vi "Main.vi"() -> (3 "Angle":dbl format="%#_4g")   [LabVIEW 2021]
doc: "The myRIO Project template acquires acceleration data from the onboard accelerometer and displays the changes of acceleration values in a waveform chart."
uses:
  <vilib>/myRIO/Instrument Drivers/Utilities/Utilities.lvlib
  <vilib>/myRIO/Express VI/Onboard IO/DO/DO Express VI.xnode
  <vilib>/myRIO/Instrument Drivers/Onboard IO/DIO/vis/Write.vi
  <vilib>/myRIO/Instrument Drivers/Onboard IO/DIO/DIO.lvlib
  <vilib>/myRIO/Common/Instrument Driver Framework/myRIO v1.0/DIO/typedefs/DIO Channels Enum.ctl
  <vilib>/myRIO/Common/Instrument Driver Framework/myRIO v1.0/DIO/typedefs/DIO Channels List.ctl
  <vilib>/myRIO/Common/Instrument Driver Framework/Utilities/typedefs/Generic FPGA Reference.ctl
  <vilib>/myRIO/Common/Instrument Driver Framework/Utilities/typedefs/myRIO v1.0 Reference.ctl
  <vilib>/myRIO/Common/Instrument Driver Framework/Utilities/typedefs/Hardware Version Enum.ctl
  <vilib>/myRIO/Common/Instrument Driver Framework/Utilities/typedefs/myRIO Generic Hardware Reference.ctl
  <vilib>/myRIO/Instrument Drivers/Onboard IO/DIO/typedefs/DIO Reference.ctl
  <vilib>/myRIO/Instrument Drivers/Onboard IO/DIO/vis/myRIO DIO Open.xnode
  <vilib>/myRIO/Common/Instrument Driver Framework/Utilities/vis/Is FPGA Ref Available.vi
  <vilib>/myRIO/Common/Instrument Driver Framework/myRIO v1.0/DIO/vis/myRIO v1.1 Open DIO.vi
  <vilib>/userdefined/High Color/nirio_resource_hc.ctl
panel:
  out "Solenoid":bool
  out "Pump":bool
  out "Angle Y":dbl format="%#_4g"
  out "Duty cycle Y":dbl format="%#_3g"
  in  "Stop Button":bool
  out "Duty cycle":dbl format="%#_3g"
  out "?":errorcluster
  # "Servo X"
  # "Servo Y"
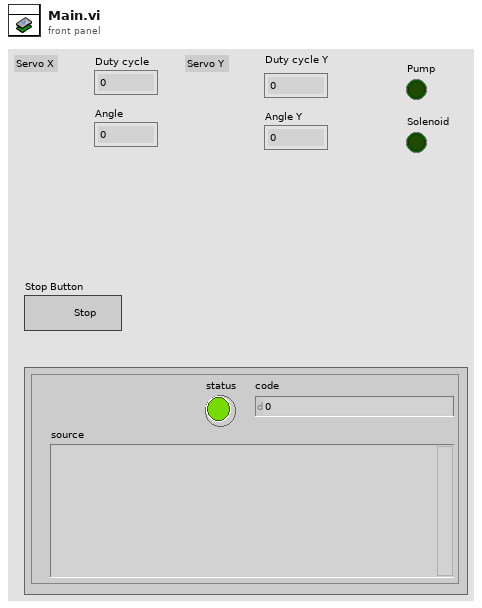
[diagram p1: front panel]
types:
  T1 = typedef "DIO.lvlib/DIO Reference.ctl" = cluster{"myRIO Reference":T2, "DIO Channels List":T6}
  T2 = typedef "myRIO Generic Hardware Reference.ctl" = cluster{"myRIO Model":T3, "myRIO Hardware Reference":T4}
  T3 = typedef "Hardware Version Enum.ctl" = enum16{"Unknown", "myRIO-1900", "myRIO-1950", "roboRIO", "NI ELVIS RIO CM", "ELVIS III"}
  T4 = typedef "myRIO v1.0 Reference.ctl" = cluster{"Generic FPGA Reference":T5, "Allow multiple opens":bool}
  T5 = typedef "Generic FPGA Reference.ctl" = refnum<k20>
  T6 = typedef "DIO Channels List.ctl" = T7[]
  T7 = typedef "DIO Channels Enum.ctl" = enum16{"Not Connected", "C/DIO0", "C/DIO1", "C/DIO2", "C/DIO3", "C/DIO4", "C/DIO5", "C/DIO6", "C/DIO7", "A/DIO0", "A/DIO1", "A/DIO2", "A/DIO3", "A/DIO4", "A/DIO5", "A/DIO6", "A/DIO7", "A/DIO8", "A/DIO9", "A/DIO10", "A/DIO11", "A/DIO12", "A/DIO13", "A/DIO14", "A/DIO15", "A/DIO16", "A/DIO17", "A/DIO18", "A/DIO19", "B/DIO0", "B/DIO1", "B/DIO2", "B/DIO3", "B/DIO4", "B/DIO5", "B/DIO6", "B/DIO7", "B/DIO8", "B/DIO9", "B/DIO10", "B/DIO11", "B/DIO12", "B/DIO13", "B/DIO14", "B/DIO15", "B/DIO16", "B/DIO17", "B/DIO18", "B/DIO19", "LED0", "LED1", "LED2", "LED3", "Button0", "DIO/DIO0", "DIO/DIO1", "DIO/DIO2", "DIO/DIO3", "DIO/DIO4", "DIO/DIO5", "DIO/DIO6", "DIO/DIO7", "DIO/DIO8", "DIO/DIO9", "SPI/CS0", "SPI/CS1", "SPI/CS2", "SPI/CS3", "LED RADIO (Green)", "LED RADIO (Red)", "LED COMM (Green)", "LED COMM (Red)", "LED MODE (Green)", "LED MODE (Red)"}
  T8 = typedef "nirio_resource_hc.ctl" = tag
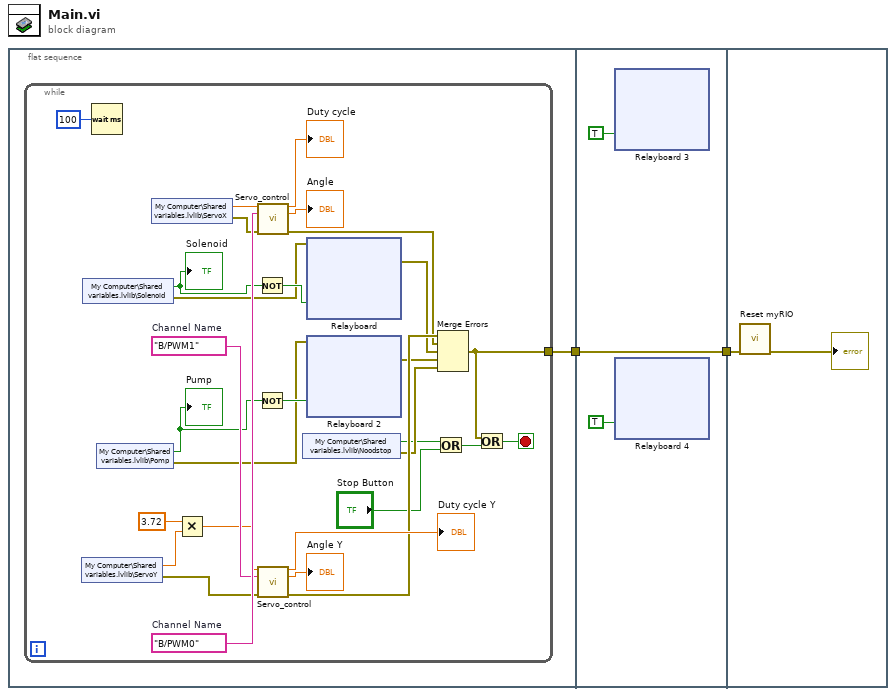
[diagram p0: block diagram]
diagram:
  n1 = flat-sequence {
    tunnel: [w3] -> w2
    tunnel: w2 -> [w105]
    tunnel: [w105] -> w1
    tunnel: w1 -> [w176]
    frame #0 {
      n2 = while {
        tunnel: [w23] -> w3
        stop <- w14 stop-if-true
        w28 = tag "B/PWM1"  # Channel Name
        w29 = tag "B/PWM0"  # Channel Name
        n3 = shared-variable "My Computer\\Shared variables.lvlib\\ServoY"() -> (w6:dbl, error out=w27:errorcluster)  [unwired: 1 in]
        n4 = shared-variable "My Computer\\Shared variables.lvlib\\Solenoid"() -> (w17:bool, error out=w13:errorcluster)  [unwired: 1 in]
        "Solenoid" <- w17
        n5 = Wait (ms)(milliseconds to wait=u32 100 ("millisecond timer value")) -> ()  [unwired: 1 out]
        n6 = shared-variable "My Computer\\Shared variables.lvlib\\Pomp"() -> (w19:bool, error out=w12:errorcluster)  [unwired: 1 in]
        "Pump" <- w19
        n7 = shared-variable "My Computer\\Shared variables.lvlib\\ServoX"() -> (w7:dbl, error out=w8:errorcluster)  [unwired: 1 in]
        n8 = Multiply(x=3.72, y=w6) -> (x*y=w5:dbl)
        n9 = Not(x=w17) -> (.not. x?=w16:bool)
        n10 = Not(x=w19) -> (.not. x?=w18:bool)
        n11 = call "Servo_control.vi"("Slide in"=w7, "Channel Name"=w29, "error in (no error)"=w8) -> ("Duty cycle"=→"Duty cycle":dbl, "Angle"=→"Angle":dbl, "error out"=w22:errorcluster)  [unwired: 10 in]
        n12 = call "Servo_control.vi"("Slide in"=w5, "Channel Name"=w28, "error in (no error)"=w27) -> ("Duty cycle"=→"Duty cycle Y":dbl, "Angle"=→"Angle Y":dbl, "error out"=w24:errorcluster)  [unwired: 10 in]
        n13 = shared-variable "My Computer\\Shared variables.lvlib\\Noodstop"() -> (w11:bool, error out=w15:errorcluster)  [unwired: 1 in]
        n14 = xnode "Relayboard"("B/DIO15 (Pin 34)"=w16, "error in (no error)"=w13) -> ("error out"=w21:errorcluster)
        n15 = xnode "Relayboard 2"("B/DIO14 (Pin 32)"=w18, "error in (no error)"=w12) -> ("error out"=w20:errorcluster)
        n16 = Or(x=w11, y="Stop Button") -> (x .or. y?=w9:bool)
        n17 = Merge Errors(w24, w22, w21, w20, w15) -> (w23:errorcluster)
        n18 = Or(x=w23, y=w9) -> (x .or. y?=w14:bool)
      }
    }
    frame #1 {
      n19 = xnode "Relayboard 3"("B/DIO15 (Pin 34)"=TRUE) -> ()  [unwired: 1 in, 1 out]
      n20 = xnode "Relayboard 4"("B/DIO14 (Pin 32)"=TRUE) -> ()  [unwired: 1 in, 1 out]
    }
    frame #2 {
      n21 = call <vilib>:"Reset myRIO.vi"("error in (no error)"=w176) -> ("error out"=→"?":errorcluster)  [unwired: 10 in]
    }
  }
